vi "Stop.vi"(8 "error in":errorcluster, 11 "NEO480 in":refnum<class "Virtual Thermometer.lvclass">) -> (0 "error out":errorcluster, 3 "NEO480 out":refnum<class "Virtual Thermometer.lvclass">)   [LabVIEW 2024, in "Virtual Thermometer.lvclass"]
uses:
  Virtual Thermometer.lvclass
  Interfaces/IRunnable/IRunnable.lvclass
  Virtual Thermometer.lvclass/Virtual Thermometer.ctl
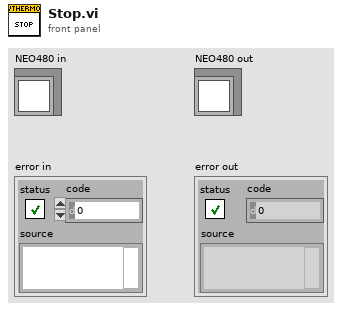
[diagram p1: front panel]
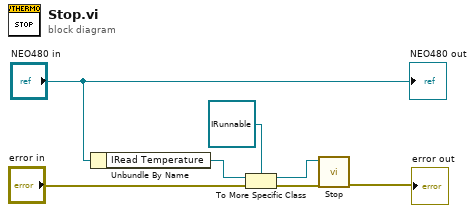
[diagram p0: block diagram]
diagram:
  n1 = Unbundle By Name("NEO480 in") -> ("IRead Temperature"=w3:refnum<class "IRead Temperature.lvclass">)
  n2 = To More Specific Class(target class=refnum<class "IRunnable.lvclass"> refnum ("IRunnable.lvclass"), reference=w3, error in="error in") -> (specific class reference=w2:refnum<class "IRunnable.lvclass">, error out=w4:errorcluster)
  n3 = call-dynamic "Stop.vi"("error in"=w4, "IRunnable in"=w2) -> ("error out"=→"error out":errorcluster)  [unwired: 8 in, 1 out]
  "NEO480 out" <- "NEO480 in"
